vi "SunVI_Complementary_Filter.vi"(9 "Gryo Displacement":dbl[](array[numeric]), 11 "Linear Acceleration":dbl[](array[numeric])) -> ()   [LabVIEW 2014]
uses:
  Globals_Real.vi
panel:
  out "s? t:f":dbl
  out "x+y":dbl
  out "In Range?":bool
  out "Accel Magnitude":dbl
  # "Complentary FilTaH"
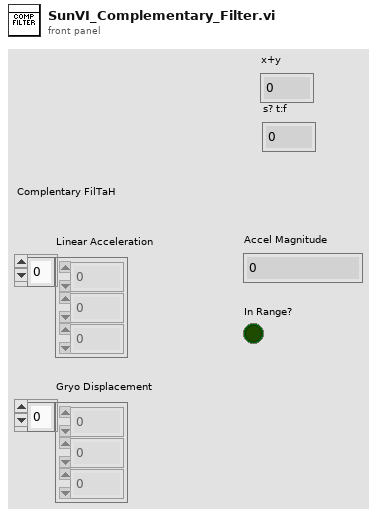
[diagram p1: front panel]
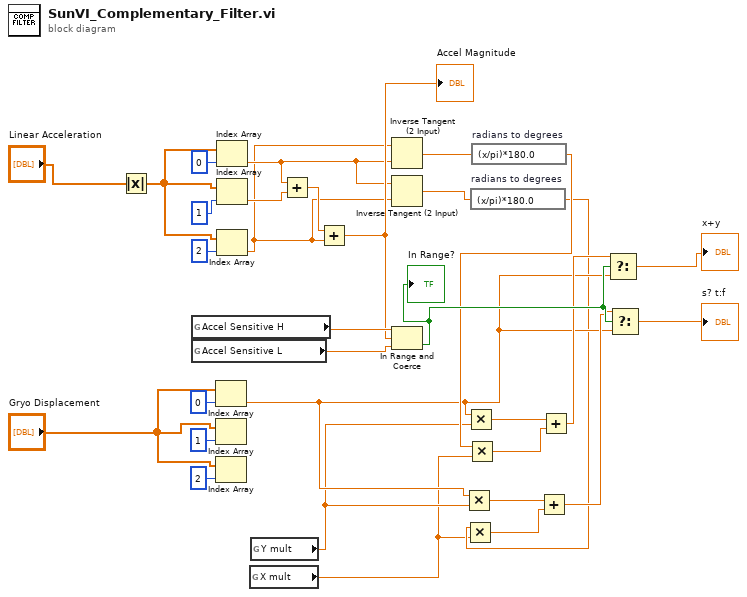
[diagram p0: block diagram]
diagram:
  n1 = Absolute Value(x="Linear Acceleration") -> (abs(x)=w26:dbl[])
  n2 = global read "Globals_Real.vi" "Accel Sensitive H"() -> (w25:dbl)
  n3 = global read "Globals_Real.vi" "Accel Sensitive L"() -> (w24:dbl)
  n4 = Index Array(array="Gryo Displacement", index=0) -> (element=w4:dbl)
  n5 = Index Array(array="Gryo Displacement", index=1) -> ()  [unwired: 1 out]
  n6 = Index Array(array="Gryo Displacement", index=2) -> ()  [unwired: 1 out]
  n7 = Index Array(array=w26, index=0) -> (element=w16:dbl)
  n8 = Index Array(array=w26, index=1) -> (element=w28:dbl)
  n9 = Index Array(array=w26, index=2) -> (element=w15:dbl)
  n10 = global read "Globals_Real.vi" "X mult"() -> (w1:dbl)
  n11 = global read "Globals_Real.vi" "Y mult"() -> (w2:dbl)
  n12 = Add(x=w16, y=w28) -> (x+y=w29:dbl)
  n13 = Add(x=w29, y=w15) -> (x+y=w23:dbl)
  "Accel Magnitude" <- w23
  n14 = Inverse Tangent (2 Input)(1:w16, 2:w15) -> (0:w18:dbl)
  n15 = Inverse Tangent (2 Input)(1:w15, 2:w16) -> (0:w17:dbl)
  n16 = In Range and Coerce(upper limit=w25, x=w23, lower limit=w24) -> (In Range?=w14:bool)  [unwired: 1 out]
  "In Range?" <- w14
  n17 = Multiply(x=w4, y=w2) -> (x*y=w7:dbl)
  n18 = Multiply(x=w4, y=w2) -> (x*y=w13:dbl)
  n19 = expression code="(x/pi)*180.0" "radians to degrees"(w17) -> (w3:dbl)
  n20 = Multiply(x=w3, y=w1) -> (x*y=w8:dbl)
  n21 = expression code="(x/pi)*180.0" "radians to degrees"(w18) -> (w9:dbl)
  n22 = Multiply(x=w9, y=w1) -> (x*y=w12:dbl)
  n23 = Add(x=w7, y=w8) -> (x+y=w6:dbl)
  n24 = Add(x=w13, y=w12) -> (x+y=w11:dbl)
  n25 = Select(t=w11, s=w14, f=w4) -> (s? t:f=→"x+y":dbl)
  n26 = Select(t=w6, s=w14, f=w4) -> (s? t:f=→"s? t:f":dbl)
